vi "GetMeasurementValues.vi"(8 "Error in":errorcluster, 9 "Index":i32, 10 "DaqMeasurement":refnum<k24>, 11 "DevicesAndSignals":T1) -> (0 "Error out":errorcluster, 1 "Waveform":waveform(dbl) caption="MeasurementValues(Waveform)", 2 "DaqMeasurement":refnum<k24>, 3 "DevicesAndSignals":T1)   [LabVIEW 2016]
doc: "Delivers measurement values in a standard LabVIEW format ( first timestamp of the measurement values in utc time format, the samplerate in 1/samplerate in Hz, and an array of measurement values).\n\nDaqMeasurement: Reference to the DaqMeasurement instance\nIndex: The index of the singnal within the given array of signals from which the measurement values should be delivered."
panel:
  out "Numerisch":dbl
  out "Zeitstempel":timestamp
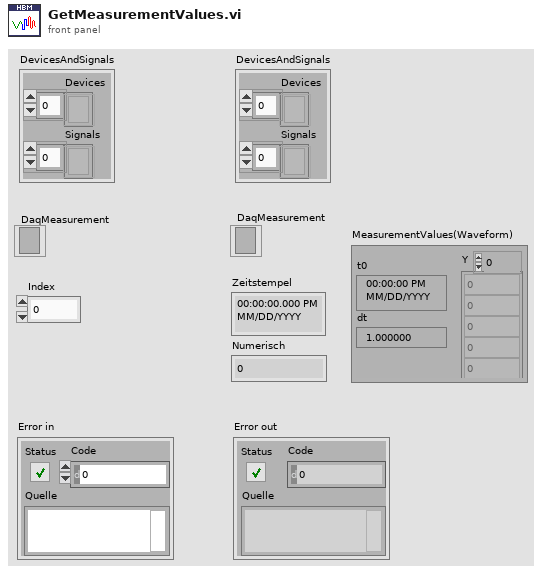
[diagram p1: front panel]
types:
  T1 = cluster{"Devices":refnum<k24>[], "Signals":refnum<k24>[]}
  T2 = typedef "LVDateTimeRec.ctl" = cluster{"Sekundenbruchteil":dbl, "Sekunde":i32, "Minute":i32, "Stunde":i32, "Tag des Monats":i32, "Monat":i32, "Jahr":i32, "Wochentag":i32, "Tag des Jahres":i32, "DST":i32}
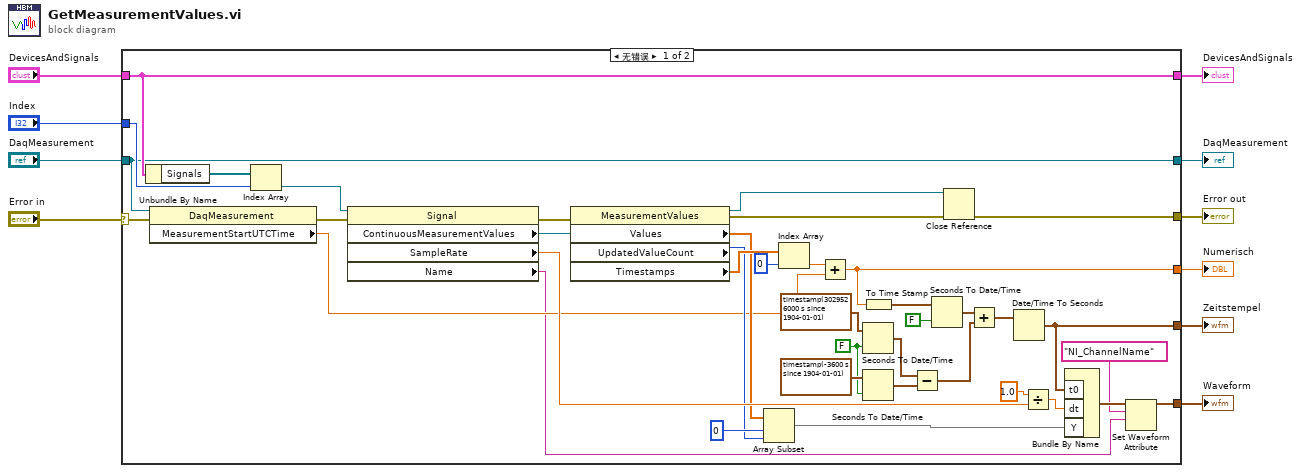
[diagram p0: block diagram]
diagram:
  n1 = case shown="无错误" "Error in" {
    selector: "Error in" -> [w21 w52]
    tunnel: "DaqMeasurement" -> [w36 w50]
    tunnel: "DevicesAndSignals" -> [w49 w51]
    tunnel: [w12 w52] -> w7
    tunnel: [w49 w51] -> w6
    tunnel: [w36 w50] -> w5
    tunnel: "Index" -> [w47 _]
    tunnel: [w18 _] -> w3
    tunnel: [w25 _] -> w2
    tunnel: [w33 _] -> w1
    frame No Error {
      w30 = FALSE ("in Weltzeit (F)")
      n2 = Unbundle By Name(w49) -> ("Signals"=w48:refnum<k24>[])
      n3 = property on="Eigenschaftsknoten" class="DaqMeasurement"(reference=w36, error in=w21) -> (error out=w20:errorcluster, "MeasurementStartUTCTime"=w34:dbl)  [unwired: 1 out]
      n4 = Index Array(array=w48, index=w47) -> (element=w14:refnum<k24>)
      n5 = property on="Eigenschaftsknoten" class="Signal"(reference=w14, error in=w20) -> (error out=w46:errorcluster, "ContinuousMeasurementValues"=w13:refnum<k24>, "SampleRate"=w43:dbl, "Name"=w17:string)  [unwired: 1 out]
      n6 = property on="Eigenschaftsknoten" class="MeasurementValues"(reference=w13, error in=w46) -> (reference out=w11:refnum<k24>, error out=w15:errorcluster, "Values"=w40:dbl[], "UpdatedValueCount"=w38:i32, "Timestamps"=w45:dbl[])
      n7 = Array Subset(array=w40, index=0 ("Index"), length=w38) -> (w37:dbl[])
      n8 = Index Array(array=w45, index=0 ("Index")) -> (element=w35:dbl)
      n9 = Add(x=w35, y=w34) -> (x+y=w33:dbl)
      n10 = Seconds To Date/Time(time stamp (now)=timestamp(3029526000 s since 1904-01-01), to UTC (F)=w30) -> (date time rec=w22:T2)
      n11 = Seconds To Date/Time(time stamp (now)=timestamp(-3600 s since 1904-01-01), to UTC (F)=w30) -> (date time rec=w23:T2)
      n12 = To Time Stamp(1:w33) -> (0:w29:timestamp)
      n13 = Subtract(x=w22, y=w23) -> (x-y=w27:T2)
      n14 = Seconds To Date/Time(time stamp (now)=w29, to UTC (F)=FALSE ("in Weltzeit (F)")) -> (date time rec=w28:T2)
      n15 = Close Reference(reference=w11, error in (no error)=w15) -> (error out=w12:errorcluster)
      n16 = Add(x=w28, y=w27) -> (x+y=w26:T2)
      n17 = Date/Time To Seconds(2:w26) -> (0:w25:timestamp)  [unwired: 1 in]
      n18 = Divide(x=1.0, y=w43) -> (x/y=w41:dbl)
      n19 = Bundle By Name("t0"=w25, "dt"=w41, "Y"=w37) -> (w19:waveform(dbl))  [unwired: 1 in]
      n20 = Set Waveform Attribute(5:w17, 6:"NI_ChannelName" ("Channel Name"), 7:w19) -> (3:w18:waveform(dbl))  [unwired: 1 in, 2 out]
    }
    frame Error {
    }
  }
  "Error out" <- w7
  "DevicesAndSignals" <- w6
  "DaqMeasurement" <- w5
  "Waveform" <- w3
  "Zeitstempel" <- w2
  "Numerisch" <- w1
